vi "Drop Message Core.vi"(11 "Execute Write Request Msg in":refnum<class "Execute Write Request Msg.lvclass">) -> ()   [LabVIEW 2020, in "PersitantConnectionHandler.lvlib" / "Execute Write Request Msg.lvclass"]
doc: "(<B>Filename</B>: Actor Framework.lvlib:Message.lvclass:Drop Message Core.vi)\n\nDefines what a message does if it is in the message queue when the queue is released. At this point, the actor has shut down, so it will never process the message.\n\nBy default, this method does nothing. A child class may override it to define behavior. National Instruments provides the Reply Msg class to override this method. This class releases its internal queue, which causes any caller of the Send Message and Wait For Response method to stop waiting and return an error."
uses:
  <vilib>/gpm_packages/@cs/Network-interface/Source/PersistantConnectionHandler/PersistantConnectionHandler Messages/Execute Write Request Msg/Execute Write Request Msg.lvclass
  <vilib>/gpm_packages/@cs/Network-interface/Source/PersistantConnectionHandler/PersistantConnectionHandler Messages/Execute Write Request Msg/Execute Write Request Msg.lvclass/Execute Write Request Msg.ctl
  <vilib>/gpm_packages/@cs/Network-interface/Source/MessagingInterfaces/WriteRequest/WriteRequest.lvclass
  <vilib>/ErrorRing/Error Ring.xnode
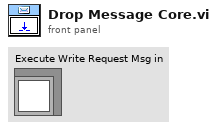
[diagram p1: front panel]
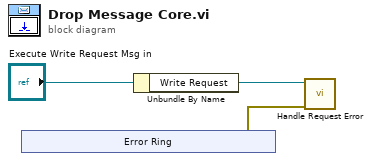
[diagram p0: block diagram]
diagram:
  n1 = xnode "Error Ring"() -> ("error out"=w1:errorcluster)
  n2 = Unbundle By Name("Execute Write Request Msg in") -> ("Write Request"=w2:refnum<class "WriteRequest.lvclass">)
  n3 = call-dynamic "Handle Request Error.vi"("Request Error"=w1, "WriteRequest in"=w2) -> ()  [unwired: 10 in]
